vi "AWS-S3-ClientRef-Get.vi"(11 "AWS-S3-API":refnum<class "AWS-S3-API.lvclass">) -> (0 "S3 Client ref":refnum<k24>, 3 "AWS-S3-API out":refnum<class "AWS-S3-API.lvclass">)   [LabVIEW 2012, in "AWS-S3-API.lvclass"]
uses:
  AWS-S3-API.lvclass
  C:/Users/Jack/repo/aws/AWS-SDK/AWSSDK.dll
  repo/aws/AWS-SDK/AWSSDK.dll
panel:
  # "Inputs"
  # "Outputs"
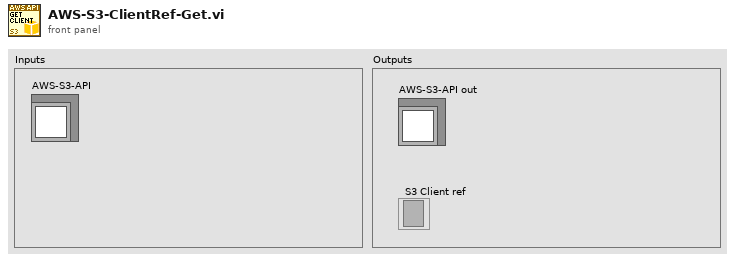
[diagram p1: front panel]
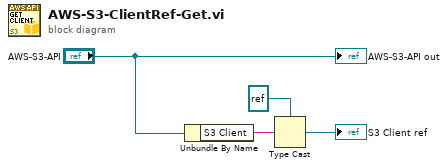
[diagram p0: block diagram]
diagram:
  n1 = Unbundle By Name("AWS-S3-API") -> ("S3 Client"=w2:string)
  n2 = Type Cast(type=refnum<k24> refnum ("S3 Client ref"), x=w2) -> (*(type *) &x=→"S3 Client ref":refnum<k24>)
  "AWS-S3-API out" <- "AWS-S3-API"
